vi "dataFiltering.vi"() -> ()   [LabVIEW 2017]
panel:
  in  "Degree":i32
  in  "GivenValue":dbl
  out "lessThanGivenValue":bool
  out "inRange_rawData":bool
  out "inRange_avgData":bool
  in  "lowRange_avgData":dbl
  in  "highRange_avgData":dbl
  in  "lowRange_data":dbl
  in  "highRange_data":dbl
  out "diff_AvgRaw":dbl
  out "exAvg_data":dbl
  out "rawData":dbl
  in  "stop":bool
  out "Waveform Chart":cluster{"number: 0 to 1":dbl, dbl}(graph)
  # "test"
  # "Low degree provides\ncloser fit between \nfiltered and raw data"
  # "*also degree\nof 0 gives\nan error"
  # "At some point I want\nto use this \"given value\"\nto determine degree\nof incoming data"
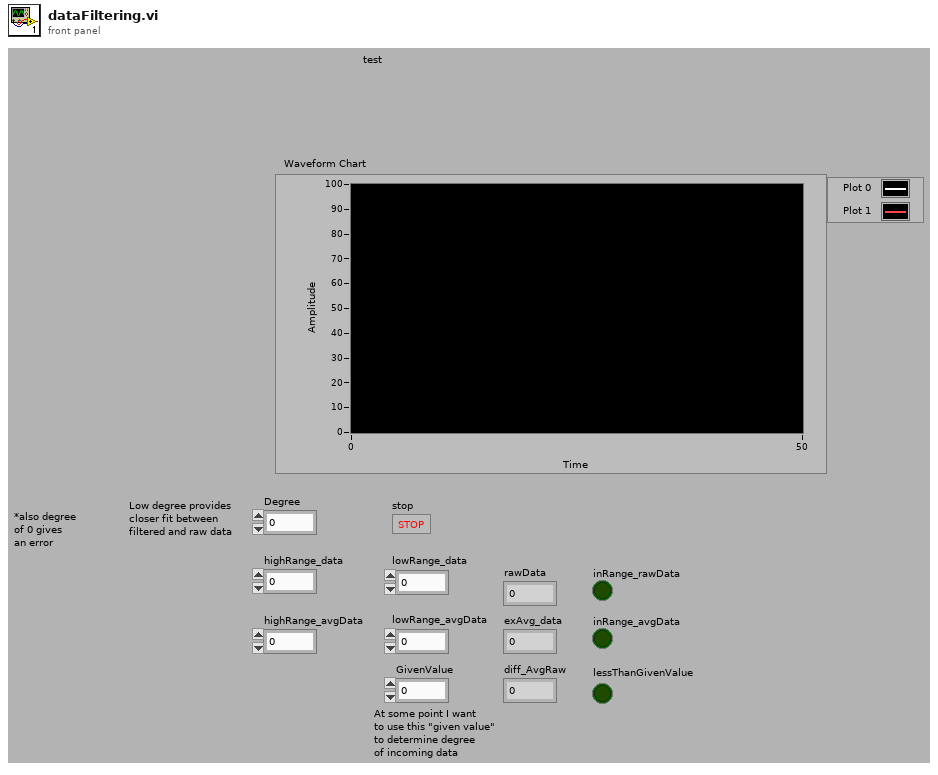
[diagram p1: front panel]
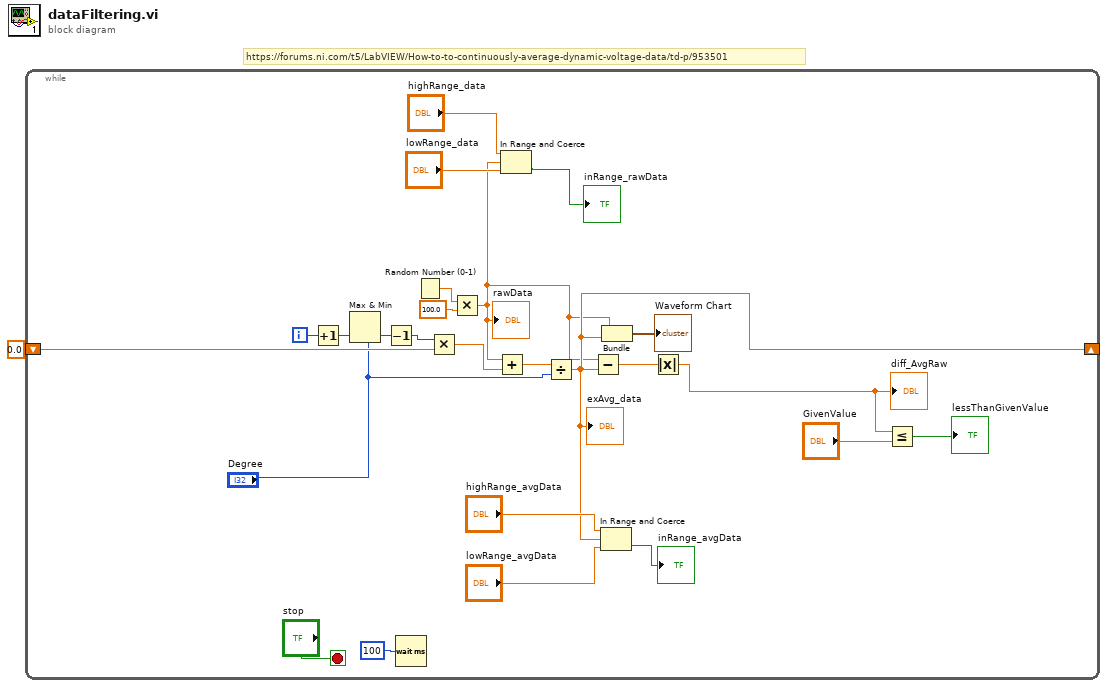
[diagram p0: block diagram]
diagram:
  # "https://forums.ni.com/t5/LabVIEW/How-to-to-continuously-average-dynamic-voltage-data/td-p/953501"
  n1 = while {
    shift-right: [w11] -> _
    shift-left: 0.0 -> [w25]
    i -> [w19]
    stop <- "stop" stop-if-true
    n2 = Increment(x=w19) -> (x+1=w18:i32)
    n3 = Max & Min(x="Degree", y=w18) -> (min(x,y)=w17:i32)  [unwired: 1 out]
    n4 = Decrement(x=w17) -> (x-1=w26:i32)
    n5 = Wait (ms)(milliseconds to wait=u32 100) -> ()  [unwired: 1 out]
    n6 = Random Number (0-1)() -> (number: 0 to 1=w14:dbl)
    n7 = Multiply(x=w26, y=w25) -> (x*y=w23:dbl)
    n8 = Multiply(x=w14, y=100.0) -> (x*y=w8:dbl)
    "rawData" <- w8
    n9 = Add(x=w8, y=w23) -> (x+y=w24:dbl)
    n10 = In Range and Coerce(upper limit="highRange_data", x=w8, lower limit="lowRange_data") -> (In Range?=→"inRange_rawData":bool)  [unwired: 1 out]
    n11 = Divide(x=w24, y="Degree") -> (x/y=w11:dbl)
    "exAvg_data" <- w11
    n12 = Subtract(x=w8, y=w11) -> (x-y=w15:dbl)
    n13 = In Range and Coerce(upper limit="highRange_avgData", x=w11, lower limit="lowRange_avgData") -> (In Range?=→"inRange_avgData":bool)  [unwired: 1 out]
    n14 = Bundle(w8, w11) -> (→"Waveform Chart":cluster{dbl, dbl})  [unwired: 1 in]
    n15 = Absolute Value(x=w15) -> (abs(x)=w4:dbl)
    "diff_AvgRaw" <- w4
    n16 = Less Or Equal?(x=w4, y="GivenValue") -> (x <= y?=→"lessThanGivenValue":bool)
  }
